vi "Properties_Get Properties From Property Node.vi"(11 "Property in":refnum<vi>) -> (3 "All Properties for Refnum Terminal":T1(array[cluster]))   [LabVIEW 2023]
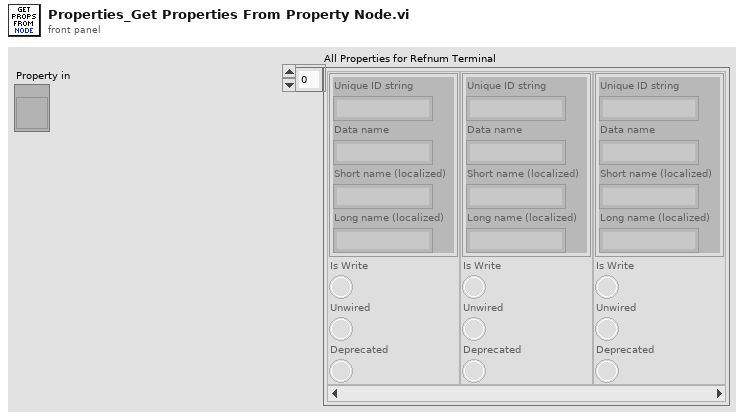
[diagram p1: front panel]
types:
  T1 = cluster{"Property/Method Info":cluster{"Unique ID string":string, "Data name":string, "Short name (localized)":string, "Long name (localized)":string}, "Is Write":bool, "Unwired":bool, "Deprecated":bool}[]
  T2 = typedef "ASPM_ArrayOfUniqueIDStringDatanameShortnameLongname.ctl" = T3[]
  T3 = typedef "ASPM_UniqueIDStringDatanameShortnameLongname.ctl" = cluster{"Unique ID string":string, "Data name":string, "Short name (localized)":string, "Long name (localized)":string}
  T4 = cluster{"Property/Method Info":cluster{"Unique ID string":string, "Data name":string, "Short name (localized)":string, "Long name (localized)":string}, "Is Write":bool, "Unwired":bool, "Deprecated":bool}
  T5 = cluster{"Unique ID string":string, "Data name":string, "Short name (localized)":string, "Long name (localized)":string}
  T6 = cluster{"Undotted Property":string, "Bare Property":string, "Is dotted?":bool, "Dot depth":i32, "Indent":i32, "Property Hierarchy":string[], "Parents":string[]}
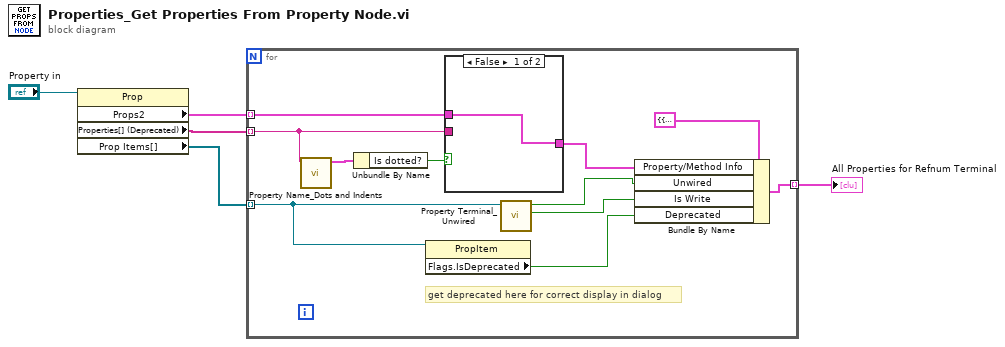
[diagram p0: block diagram]
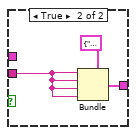
[diagram p2: hidden frame]
diagram:
  n1 = property class="Prop"(reference="Property in") -> ("Props2"=w1:T2, "Properties[] (Deprecated)"=w4:string[], "Prop Items[]"=w5:refnum<vi>[])  [unwired: 1 in, 2 out]
  n2 = for {
    tunnel: w5 -> [w11] mode=indexing
    tunnel: w4 -> [w9] mode=indexing
    tunnel: [w15] -> w2 mode=indexing
    tunnel: w1 -> [w7] mode=indexing
    # "get deprecated here for correct display in dialog"
    n3 = call "Property Name_Dots and Indents.vi"("Property"=w9) -> ("Cluster"=w10:T6)  [unwired: 10 in]
    n4 = Unbundle By Name(w10) -> ("Is dotted?"=w8:bool)
    n5 = property class="PropItem"(reference=w11) -> ("Flags.IsDeprecated"=w6:bool)  [unwired: 1 in, 2 out]
    n6 = case shown="False" w8 {
      tunnel: [w17 w20] -> w13
      tunnel: w9 -> [_ w18]
      tunnel: w7 -> [w17 _]
      frame False {
      }
      frame True {
        n7 = Bundle(cluster=T5 {"Unique ID string"="", "Data name"="", "Short name (localized)"="", "Long name (localized)"=""} ("Property/Method Info"), "Unique ID string"=w18, "Data name"=w18, "Short name (localized)"=w18, "Long name (localized)"=w18) -> (w20:T5)
      }
    }
    n8 = call "Property Terminal_Unwired.vi"("PropertyItem in"=w11) -> ("Is Write"=w12:bool, "Unwired"=w14:bool)  [unwired: 8 in, 1 out]
    n9 = Bundle By Name(cluster=T4 {"Property/Method Info"={"Unique ID string"="", "Data name"="", "Short name (localized)"="", "Long name (localized)"=""}, "Is Write"=FALSE, "Unwired"=FALSE, "Deprecated"=FALSE} ("Cluster"), "Property/Method Info"=w13, "Unwired"=w14, "Is Write"=w12, "Deprecated"=w6) -> (w15:T4)
  }
  "All Properties for Refnum Terminal" <- w2
